vi "Insert bitt error in string.vi"(1 "Fault(fraction = 0)":dbl, 7 "Transmitt string":string) -> (8 "string with bit errors":string)   [LabVIEW 2011]
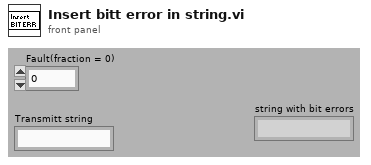
[diagram p1: front panel]
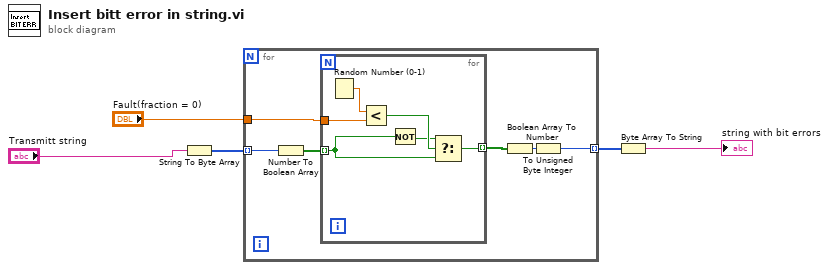
[diagram p0: block diagram]
diagram:
  n1 = String To Byte Array(string="Transmitt string") -> (unsigned byte array=w2:u8[])
  n2 = for {
    tunnel: w2 -> [w11] mode=indexing
    tunnel: "Fault(fraction = 0)" -> [w9]
    tunnel: [w6] -> w4 mode=indexing
    n3 = Number To Boolean Array(number=w11) -> (Boolean array=w10:bool[])
    n4 = for {
      tunnel: w10 -> [w13] mode=indexing
      tunnel: w9 -> [w16]
      tunnel: [w12] -> w8 mode=indexing
      n5 = Random Number (0-1)() -> (number: 0 to 1=w17:dbl)
      n6 = Less?(x=w17, y=w16) -> (x < y?=w15:bool)
      n7 = Not(x=w13) -> (.not. x?=w14:bool)
      n8 = Select(t=w14, s=w15, f=w13) -> (s? t:f=w12:bool)
    }
    n9 = Boolean Array To Number(Boolean array=w8) -> (number=w7:u32)
    n10 = To Unsigned Byte Integer(number=w7) -> (unsigned 8bit integer=w6:u8)
  }
  n11 = Byte Array To String(unsigned byte array=w4) -> (string=→"string with bit errors":string)
